vi "TDMS Reader.vi"   [LabVIEW 2016]
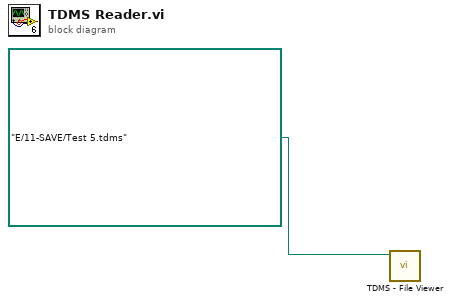
[diagram p0: block diagram]
diagram:
  n1 = call <vilib>:"TDMS - File Viewer.vi"("file path"=path "E:/11-SAVE/Test 5.tdms") -> ()  [unwired: 5 in, 2 out]
